vi "GetIntArrTo1DimenArrayCtrl.vi"(11 "array in":refnum<vi>) -> (2 "array data":i32[](array[numeric]), 3 "array out":refnum<vi>)   [LabVIEW 2018, in "Library-Ctrl.lvlib"]
uses:
  Library-Ctrl.lvlib
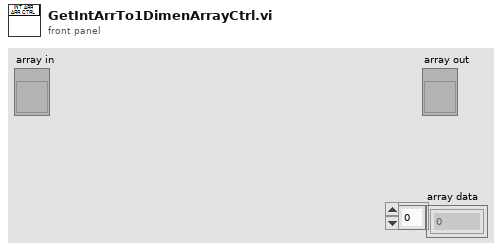
[diagram p1: front panel]
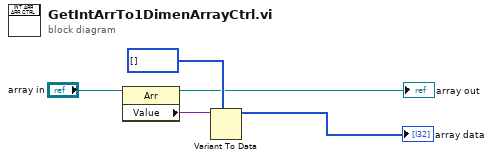
[diagram p0: block diagram]
diagram:
  n1 = property class="Arr"(reference="array in") -> (reference out=→"array out":refnum<vi>, "Value"=w4:variant)  [unwired: 1 in, 1 out]
  n2 = Variant To Data(type=i32[] [] ("array data"), Variant=w4) -> (data=→"array data":i32[])  [unwired: 1 in, 1 out]
